vi "LatchRefs.vi"() -> ()   [LabVIEW 2014, in "LatchLib.lvlib"]
uses:
  LatchRefs.ctl
  LatchLib.lvlib
panel:
  in  "Enum":T1
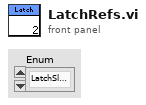
[diagram p1: front panel]
types:
  T1 = typedef "LatchLib.lvlib/LatchRefs.ctl" = enum16{"LatchSloenoid", "ContainerSolenoid"}
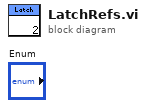
[diagram p0: block diagram]
diagram:
